vi "Tranlate points to this origin.vi"(6 "error in (no error)":errorcluster, 7 "Laser Position":cluster{"x":i16, "y":i16}={"x"=1139, "y"=846}, 8 "New Origin Point":cluster{"x":i16, "y":i16}={"x"=1139, "y"=846}, 9 "Points":cluster{"X":i32, "Y":i32}[](array[cluster])) -> (0 "error out":errorcluster, 3 "Shift points":cluster{"X":i32, "Y":i32}[](array[cluster]))   [LabVIEW 2017]
doc: "Use this template to build a VI to use as a subVI."
uses:
  <vilib>/Analysis/coordinate.llb/2D Cartesian Coordinate Shift (Array).vi
  <vilib>/Analysis/NI_AALPro.lvlib
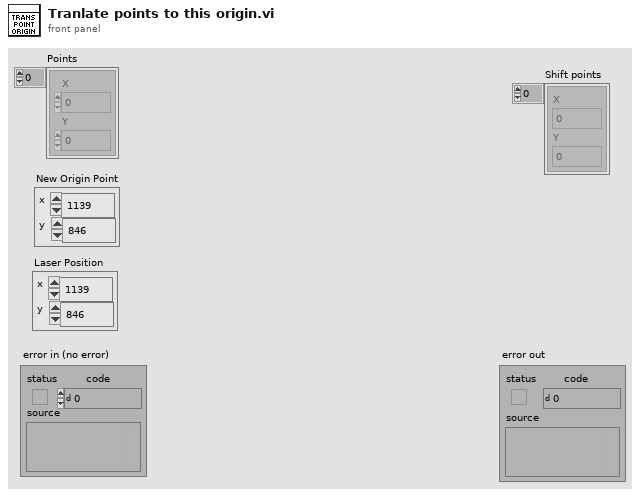
[diagram p1: front panel]
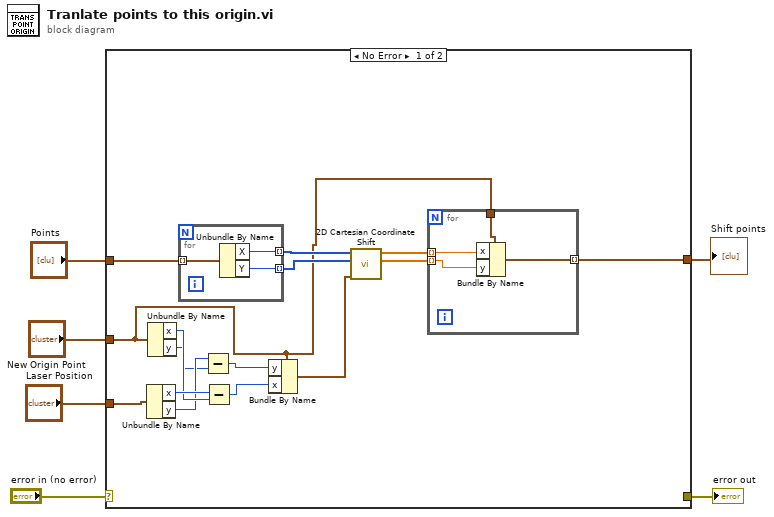
[diagram p0: block diagram]
diagram:
  n1 = case shown="No Error" "error in (no error)" {
    selector: "error in (no error)" -> [_ w30]
    tunnel: [_ w30] -> w5
    tunnel: "Points" -> [w21 w29]
    tunnel: "New Origin Point" -> [w10 _]
    tunnel: [w16 w29] -> w2
    tunnel: "Laser Position" -> [w15 _]
    frame No Error {
      n2 = Unbundle By Name(w15) -> ("x"=w14:i16, "y"=w12:i16)
      n3 = Unbundle By Name(w10) -> ("x"=w13:i16, "y"=w11:i16)
      n4 = for {
        tunnel: w21 -> [w28] mode=indexing
        tunnel: [w27] -> w20 mode=indexing
        tunnel: [w26] -> w19 mode=indexing
        n5 = Unbundle By Name(w28) -> ("X"=w27:i32, "Y"=w26:i32)
      }
      n6 = Subtract(x=w12, y=w11) -> (x-y=w9:i16)
      n7 = Subtract(x=w14, y=w13) -> (x-y=w8:i16)
      n8 = Bundle By Name(cluster=w10, "y"=w9, "x"=w8) -> (w7:cluster{"x":i16, "y":i16})
      n9 = call-poly <vilib>:"2D Cartesian Coordinate Shift.vi"("shift"=w7, "Y"=w19, "X"=w20) -> ("Y Out"=w17:dbl[], "X Out"=w18:dbl[])  [unwired: 6 in, 1 out]
      n10 = for {
        tunnel: w18 -> [w24] mode=indexing
        tunnel: w17 -> [w23] mode=indexing
        tunnel: w10 -> [w25]
        tunnel: [w22] -> w16 mode=indexing
        n11 = Bundle By Name(cluster=w25, "x"=w24, "y"=w23) -> (w22:cluster{"x":i16, "y":i16})
      }
    }
    frame Error {
    }
  }
  "error out" <- w5
  "Shift points" <- w2
